vi "ZZZ Chroma 1905x Series Status-.vi"(3 "error in":T1, 5 "inst handle in":refnum<visa-resource-name>) -> (0 "error out":T1, 1 "Status":string, 2 "inst handle out":refnum<visa-resource-name>)   [LabVIEW 2025]
panel:
  # "Status?"
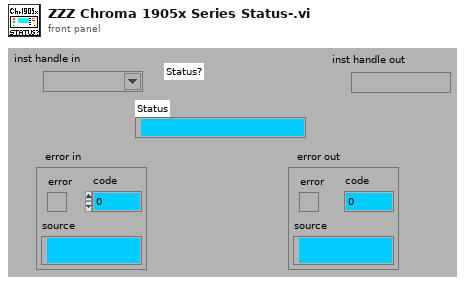
[diagram p1: front panel]
types:
  T1 = cluster{"error":bool, "code":i8, "source":string}
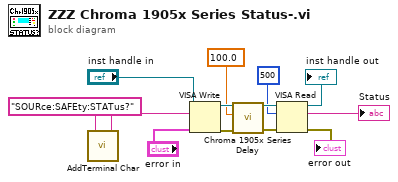
[diagram p0: block diagram]
diagram:
  n1 = call "AddTerminal Char.vi"("Cmd string"="SOURce:SAFEty:STATus?") -> ("Concatenated String"=w2:string)  [unwired: 4 in]
  n2 = VISA Write(VISA resource name="inst handle in", write buffer=w2, error in (no error)="error in") -> (VISA resource name out=w8:refnum<visa-resource-name>, error out=w9:errorcluster)  [unwired: 1 out]
  n3 = call "Chroma 1905x Series Delay.vi"("error in (no error)"=w9, "Time Delay [ms]"=100.0 ("Time Delay S"), "VISA resource name"=w8) -> ("error out"=w10:errorcluster, "VISA resource name 2"=w7:refnum<visa-resource-name>)  [unwired: 7 in]
  n4 = VISA Read(VISA resource name=w7, byte count=u32 500 ("byte count (0)"), error in (no error)=w10) -> (VISA resource name out=→"inst handle out":refnum<visa-resource-name>, read buffer=→"Status":string, error out=→"error out":errorcluster)  [unwired: 1 out]
